vi "Suspend heater.vi"(8 "error in (no error)":errorcluster, 10 "Heater %":dbl=-1.0, 11 "VISA resource name":refnum<visa-resource-name>) -> (0 "error out":errorcluster, 1 "I":dbl, 2 "P":dbl, 3 "VISA resource name out":refnum<visa-resource-name>, 4 "D":dbl, 5 "P0":dbl)   [LabVIEW 2015]
uses:
  GPIB/VISA  Send Receive.vi
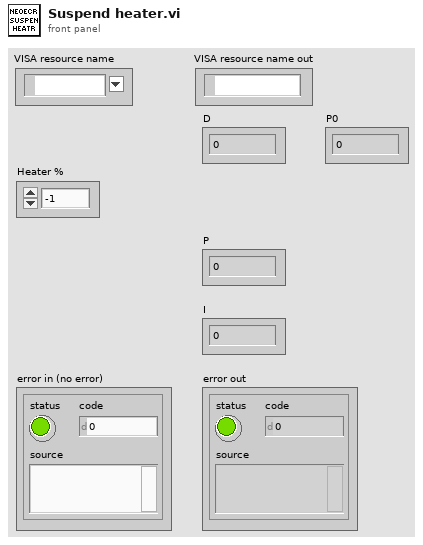
[diagram p1: front panel]
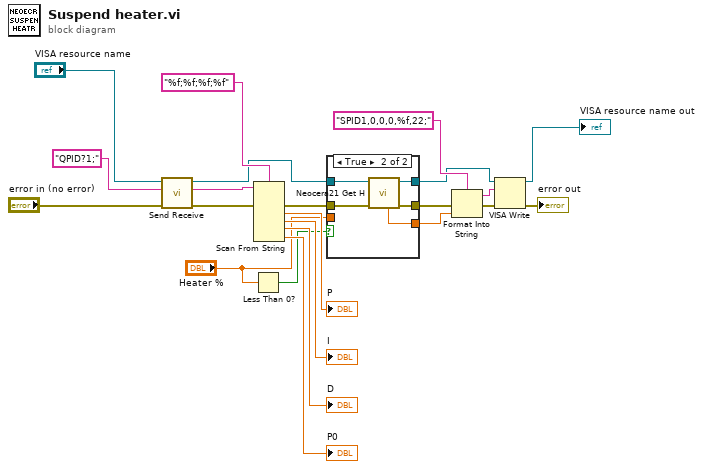
[diagram p0: block diagram]
diagram:
  n1 = call-poly "Send Receive.vi"("error in (no error)"="error in (no error)", "data string in"="QPID?1;" ("write buffer"), "VISA Resource Name"="VISA resource name") -> ("error out"=w20:errorcluster, "data string out"=w22:string, "VISA Resource Name Out"=w8:refnum<visa-resource-name>)  [unwired: 6 in]
  n2 = Less Than 0?(x="Heater %") -> (x < 0?=w9:bool)
  n3 = Scan From String(format string="%f;%f;%f;%f", input string=w22, error in=w20) -> (error out=w6:errorcluster, output 1=→"P":dbl, output 2=→"I":dbl, output 3=→"D":dbl, output 4=→"P0":dbl)  [unwired: 5 in, 2 out]
  n4 = case shown="True" w9 {
    tunnel: w8 -> [w23 w30]
    tunnel: [w23 w29] -> w7
    tunnel: w6 -> [w24 w28]
    tunnel: [w24 w27] -> w5
    tunnel: [w25 w26] -> w4
    tunnel: "Heater %" -> [w25 _]
    frame False {
    }
    frame True {
      n5 = call "Neocera21 Get H.vi"("error in (no error)"=w28, "VISA Resource Name"=w30) -> ("error out"=w27:errorcluster, "VISA Resource Name Out"=w29:refnum<visa-resource-name>, "Heat %"=w26:dbl)  [unwired: 4 in, 3 out]
    }
  }
  n6 = Format Into String(format string="SPID1,0,0,0,%f,22;", error in=w5, w4) -> (resulting string=w12:string, error out=w11:errorcluster)  [unwired: 1 in]
  n7 = VISA Write(VISA resource name=w7, write buffer=w12, error in (no error)=w11) -> (VISA resource name out=→"VISA resource name out":refnum<visa-resource-name>, error out=→"error out":errorcluster)  [unwired: 1 out]
